vi "myBOT_Create.vi"(8 "error in (no error)":errorcluster) -> (0 "error out":errorcluster, 3 "SceneObject out":refnum<vi>)   [LabVIEW 2013]
doc: "\"myBOT_Create.vi\": This VI allow to create a new 3D Robot object. This VI was developed for the myRIO Balancing Robot Project. See https://decibel.ni.com/content/groups/myrio-balancing-robot for more information and example projects."
uses:
  <vilib>/Utility/miscctls.llb/LV3DPointTypeDef.ctl
  <vilib>/picture/3D Picture Control/Object/Create Object (name).vi
  <vilib>/picture/3D Picture Control/NI_3D Picture Control.lvlib
panel:
  out "3D Picture":refnum<vi>(3d-picture)
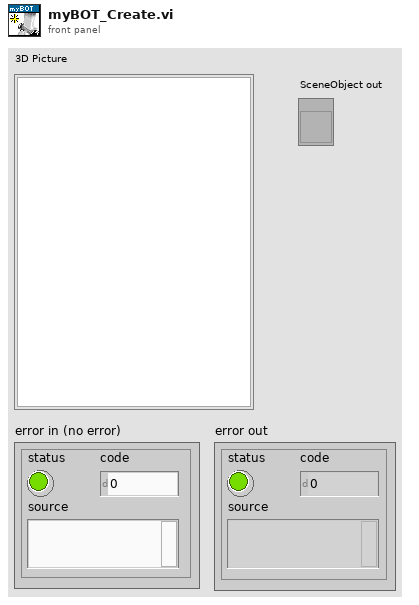
[diagram p1: front panel]
types:
  T1 = cluster{"Red":sgl, "Green":sgl, "Blue":sgl, "Alpha":sgl}
  T2 = typedef "LV3DPointTypeDef.ctl" = cluster{"X":sgl, "Y":sgl, "Z":sgl}
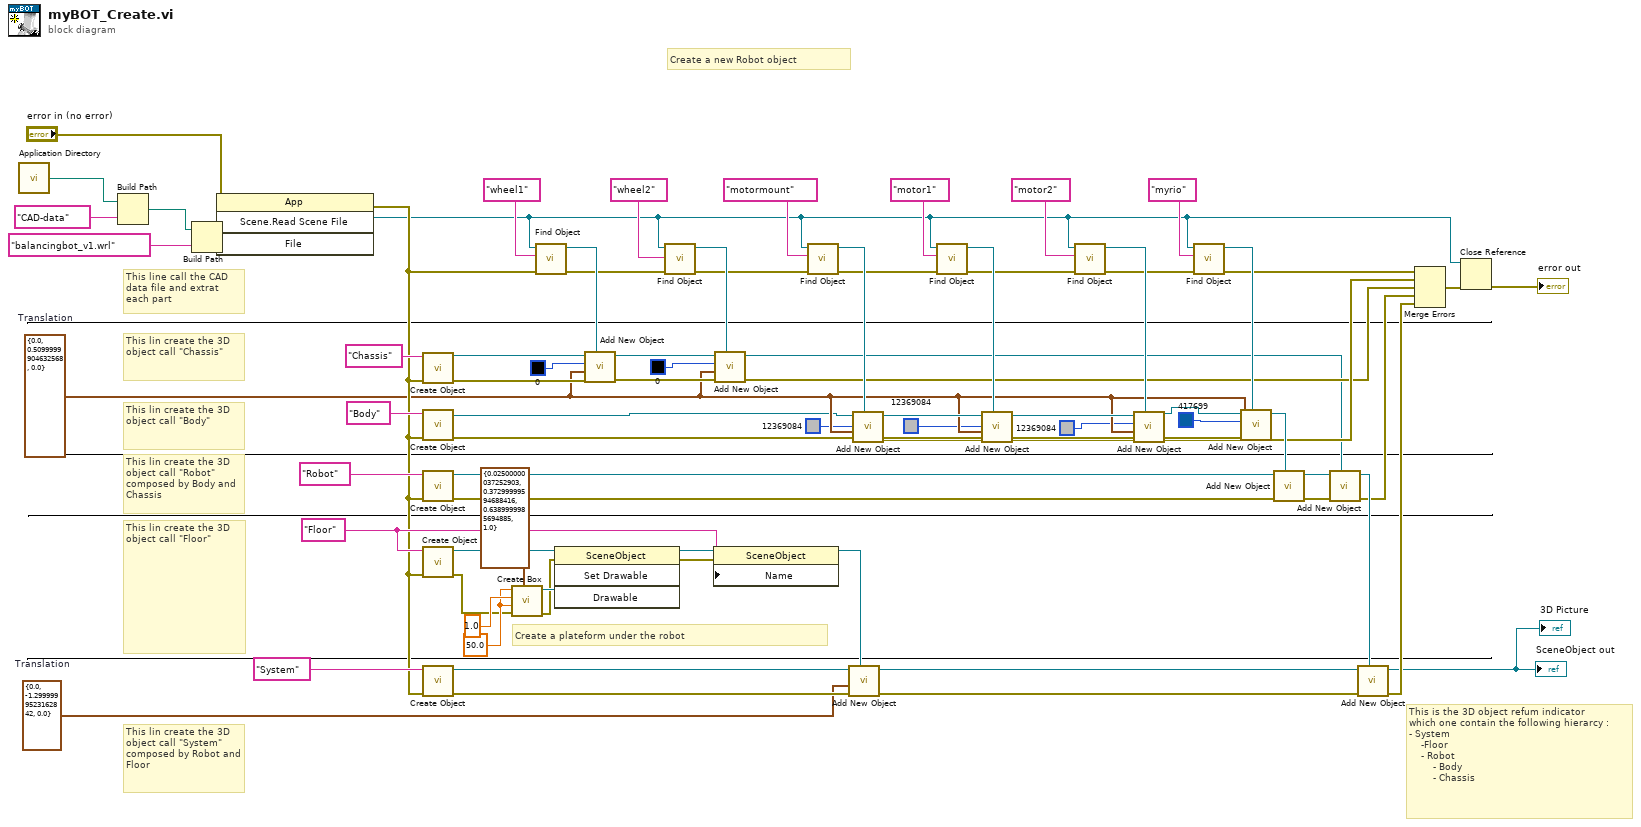
[diagram p0: block diagram]
diagram:
  w21 = T2 {"X"=0.0, "Y"=-1.3, "Z"=0.0}  # Translation
  w20 = T2 {"X"=0.0, "Y"=0.51, "Z"=0.0}  # Translation
  w50 = sgl 50.0 ("Length X")
  w44 = "Floor" ("Name")
  # "Create a plateform under the robot"
  # "Create a new Robot object"
  # "This is the 3D object refum indicator \nwhich one contain the following hierarcy :\n- System\n    -Floor\n    - Robot\n        - Body\n        - Chassis"
  # "This lin create the 3D object call \"Body\""
  # "This lin create the 3D object call \"System\" composed by Robot and Floor"
  # "This line call the CAD data file and extrat each part"
  # "This lin create the 3D object call \"Chassis\""
  # "This lin create the 3D object call \"Robot\" composed by Body and Chassis"
  # "This lin create the 3D object call \"Floor\""
  n1 = call <vilib>:"Application Directory.vi"() -> ("Application Directory"=w77:path)
  n2 = Build Path(base path=w77, name or relative path="CAD-data") -> (appended path=w74:path)
  n3 = Build Path(base path=w74, name or relative path="balancingbot_v1.wrl") -> (appended path=w75:path)
  n4 = invoke on="Invoke Node" class="App" method="Scene.Read Scene File"(error in="error in (no error)", "File"=w75) -> (error out=w22:errorcluster, "Scene.Read Scene File"=w14:refnum<vi>)  [unwired: 2 in, 2 out]
  n5 = call-poly <vilib>:"Create Object.vi"("error in (no error)"=w22, "Name"="Chassis") -> ("error out"=w33:errorcluster, "Scene:New Object"=w37:refnum<vi>)  [unwired: 8 in]
  n6 = call-poly <vilib>:"Create Object.vi"("error in (no error)"=w22, "Name"="Body") -> ("error out"=w34:errorcluster, "Scene:New Object"=w3:refnum<vi>)  [unwired: 8 in]
  n7 = call-poly <vilib>:"Create Object.vi"("error in (no error)"=w22, "Name"="Robot") -> ("error out"=w24:errorcluster, "Scene:New Object"=w57:refnum<vi>)  [unwired: 8 in]
  n8 = call-poly <vilib>:"Create Object.vi"("error in (no error)"=w22, "Name"=w44) -> ("error out"=w49:errorcluster, "Scene:New Object"=w51:refnum<vi>)  [unwired: 8 in]
  n9 = call-poly <vilib>:"Create Object.vi"("error in (no error)"=w22, "Name"="System") -> ("error out"=w23:errorcluster, "Scene:New Object"=w43:refnum<vi>)  [unwired: 8 in]
  n10 = call <vilib>:"Create Box.vi"("Color"=T1 {"Red"=0.025, "Green"=0.373, "Blue"=0.639, "Alpha"=1.0}, "error in (no error)"=w49, "Length Z"=w50, "Length Y"=sgl 1.0 ("Length Z"), "Length X"=w50) -> ("error out"=w48:errorcluster, "New Box Refnum"=w53:refnum<vi>)  [unwired: 5 in]
  n11 = call <vilib>:"Find Object.vi"("error in (no error)"=w22, "Object Name"="wheel1", "Scene Refnum"=w14) -> ("error out"=w29:errorcluster, "Object Refnum"=w63:refnum<vi>)  [unwired: 7 in]
  n12 = invoke class="SceneObject" method="Set Drawable"(reference=w51, error in=w48, "Drawable"=w53) -> (reference out=w46:refnum<vi>, error out=w45:errorcluster)  [unwired: 1 in, 2 out]
  n13 = call "Add New Object.vi"("NewObject in"=w63, "error in (no error)"=w33, "Translation"=w20, "Color"=u32 0, "Scene: Object"=w37) -> ("error out"=w32:errorcluster, "SceneObject out"=w38:refnum<vi>)  [unwired: 5 in]
  n14 = call <vilib>:"Find Object.vi"("error in (no error)"=w29, "Object Name"="wheel2", "Scene Refnum"=w14) -> ("error out"=w28:errorcluster, "Object Refnum"=w64:refnum<vi>)  [unwired: 7 in]
  n15 = property class="SceneObject"(reference=w46, error in=w45, "Name"=w44) -> (reference out=w42:refnum<vi>)  [unwired: 1 out]
  n16 = call "Add New Object.vi"("NewObject in"=w64, "error in (no error)"=w32, "Translation"=w20, "Color"=u32 0, "Scene: Object"=w38) -> ("error out"=w5:errorcluster, "SceneObject out"=w4:refnum<vi>)  [unwired: 5 in]
  n17 = call <vilib>:"Find Object.vi"("error in (no error)"=w28, "Object Name"="motormount", "Scene Refnum"=w14) -> ("error out"=w27:errorcluster, "Object Refnum"=w62:refnum<vi>)  [unwired: 7 in]
  n18 = call "Add New Object.vi"("NewObject in"=w42, "error in (no error)"=w23, "Translation"=w21, "Scene: Object"=w43) -> ("error out"=w40:errorcluster, "SceneObject out"=w41:refnum<vi>)  [unwired: 6 in]
  n19 = call "Add New Object.vi"("NewObject in"=w62, "Translation"=w20, "Color"=u32 12369084, "Scene: Object"=w3) -> ("error out"=w31:errorcluster, "SceneObject out"=w36:refnum<vi>)  [unwired: 6 in]
  n20 = call <vilib>:"Find Object.vi"("error in (no error)"=w27, "Object Name"="motor1", "Scene Refnum"=w14) -> ("error out"=w26:errorcluster, "Object Refnum"=w61:refnum<vi>)  [unwired: 7 in]
  n21 = call "Add New Object.vi"("NewObject in"=w61, "error in (no error)"=w31, "Translation"=w20, "Color"=u32 12369084, "Scene: Object"=w36) -> ("error out"=w30:errorcluster, "SceneObject out"=w35:refnum<vi>)  [unwired: 5 in]
  n22 = call <vilib>:"Find Object.vi"("error in (no error)"=w26, "Object Name"="motor2", "Scene Refnum"=w14) -> ("error out"=w25:errorcluster, "Object Refnum"=w60:refnum<vi>)  [unwired: 7 in]
  n23 = call "Add New Object.vi"("NewObject in"=w60, "error in (no error)"=w30, "Translation"=w20, "Color"=u32 12369084, "Scene: Object"=w35) -> ("error out"=w18:errorcluster, "SceneObject out"=w2:refnum<vi>)  [unwired: 5 in]
  n24 = call <vilib>:"Find Object.vi"("error in (no error)"=w25, "Object Name"="myrio", "Scene Refnum"=w14) -> ("error out"=w19:errorcluster, "Object Refnum"=w59:refnum<vi>)  [unwired: 7 in]
  n25 = call "Add New Object.vi"("NewObject in"=w59, "error in (no error)"=w34, "Translation"=w20, "Color"=u32 417699, "Scene: Object"=w2) -> ("SceneObject out"=w56:refnum<vi>)  [unwired: 5 in, 1 out]
  n26 = call "Add New Object.vi"("NewObject in"=w56, "error in (no error)"=w24, "Scene: Object"=w57) -> ("error out"=w55:errorcluster, "SceneObject out"=w54:refnum<vi>)  [unwired: 7 in]
  n27 = call "Add New Object.vi"("NewObject in"=w4, "error in (no error)"=w55, "Scene: Object"=w54) -> ("error out"=w17:errorcluster, "SceneObject out"=w39:refnum<vi>)  [unwired: 7 in]
  n28 = call "Add New Object.vi"("NewObject in"=w39, "error in (no error)"=w40, "Scene: Object"=w41) -> ("error out"=w16:errorcluster, "SceneObject out"=→"SceneObject out" →"3D Picture":refnum<vi>)  [unwired: 7 in]
  n29 = Merge Errors(w19, w18, w5, w17, w16) -> (w15:errorcluster)
  n30 = Close Reference(reference=w14, error in (no error)=w15) -> (error out=→"error out":errorcluster)
